vi "Test Queues.vi"() -> ()   [LabVIEW 2019, in "Generator.lvclass"]
uses:
  Generator.lvclass
  typedefs/Waveforms--Cluster.ctl
  <vilib>/measure/NI_MABase.lvlib
panel:
  out "# elements":i32
  out "Waveform Chart":cluster{dbl, dbl}(graph)
  in  "stop":bool
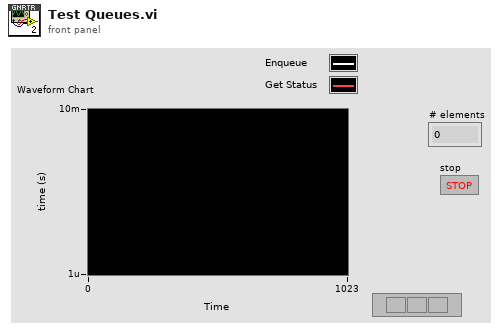
[diagram p1: front panel]
types:
  T1 = typedef "Generator.lvclass/Waveforms--Cluster.ctl" = cluster{"AO":waveform(dbl)[], "REF_X":waveform(dbl)[], "REF_Y":waveform(dbl)[]}
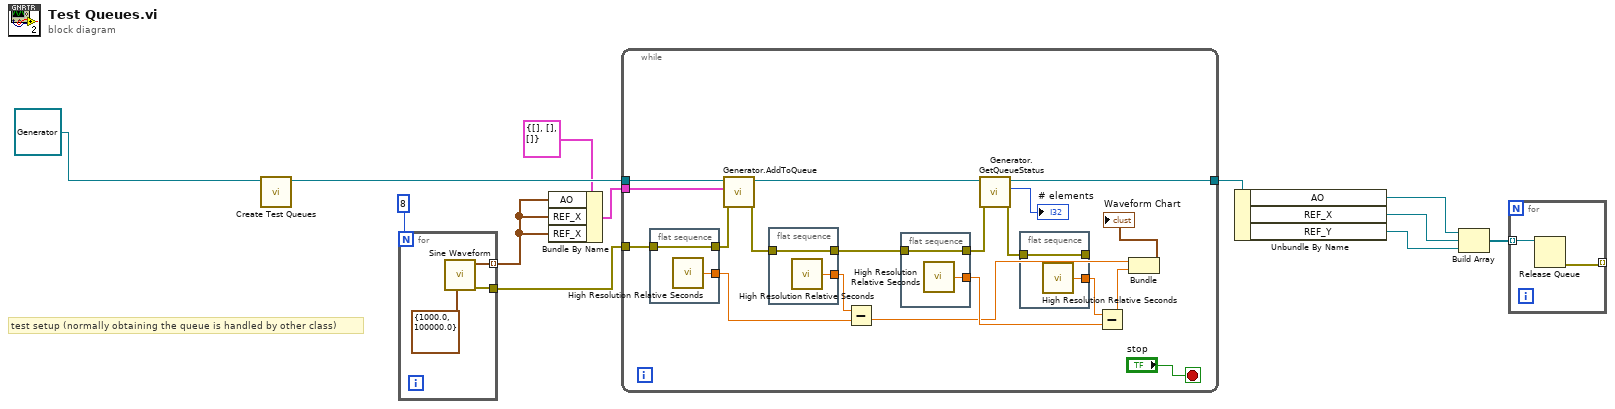
[diagram p0: block diagram]
diagram:
  # "test setup (normally obtaining the queue is handled by other class)"
  n1 = call "Create Test Queues.vi"("Generator in"=refnum<class "Generator.lvclass"> refnum ("Generator.lvclass")) -> ("Generator out"=w12:refnum<class "Generator.lvclass">)  [unwired: 10 in]
  n2 = for {
    N: 8 -> [_]
    tunnel: [w14] -> w7 mode=indexing
    tunnel: [w13] -> w8
    n3 = call <vilib>:"Sine Waveform.vi"("sampling info"=cluster{"Fs":dbl, "#s":dbl} {"Fs"=1000.0, "#s"=100000.0}) -> ("error out"=w13:errorcluster, "signal out"=w14:waveform(dbl))  [unwired: 9 in]
  }
  n4 = Bundle By Name(cluster=T1 {"AO"=[], "REF_X"=[], "REF_Y"=[]} ("Waveforms"), "AO"=w7, "REF_X"=w7, "REF_X"=w7) -> (w10:T1)
  n5 = while {
    tunnel: w12 -> [w34]
    tunnel: w10 -> [w20]
    tunnel: w8 -> [w19]
    tunnel: [w17] -> w6
    stop <- "stop" stop-if-true
    n6 = flat-sequence {
      tunnel: [w42] -> w31
      tunnel: w19 -> [w41]
      tunnel: [w41] -> w29
      frame #0 {
        n7 = call <vilib>:"High Resolution Relative Seconds.vi"() -> ("relative seconds"=w42:dbl)
      }
    }
    n8 = call "Generator.AddToQueue.vi"("error in (no error)"=w29, "Waveforms"=w20, "Generator in"=w34) -> ("error out"=w30:errorcluster, "Generator out"=w33:refnum<class "Generator.lvclass">)  [unwired: 7 in]
    n9 = flat-sequence {
      tunnel: [w40] -> w32
      tunnel: [w39] -> w25
      tunnel: w30 -> [w39]
      frame #0 {
        n10 = call <vilib>:"High Resolution Relative Seconds.vi"() -> ("relative seconds"=w40:dbl)
      }
    }
    n11 = Subtract(x=w32, y=w31) -> (x-y=w21:dbl)
    n12 = flat-sequence {
      tunnel: [w38] -> w27
      tunnel: w25 -> [w37]
      tunnel: [w37] -> w24
      frame #0 {
        n13 = call <vilib>:"High Resolution Relative Seconds.vi"() -> ("relative seconds"=w38:dbl)
      }
    }
    n14 = call "Generator.GetQueueStatus.vi"("error in (no error)"=w24, "Generator in"=w33) -> ("error out"=w23:errorcluster, "# elements"=→"# elements":i32, "Generator out"=w17:refnum<class "Generator.lvclass">)  [unwired: 7 in]
    n15 = flat-sequence {
      tunnel: [w36] -> w26
      tunnel: [w35] -> _
      tunnel: w23 -> [w35]
      frame #0 {
        n16 = call <vilib>:"High Resolution Relative Seconds.vi"() -> ("relative seconds"=w36:dbl)
      }
    }
    n17 = Subtract(x=w26, y=w27) -> (x-y=w22:dbl)
    n18 = Bundle(w21, w22) -> (→"Waveform Chart":cluster{dbl, dbl})  [unwired: 1 in]
  }
  n19 = Unbundle By Name(w6) -> ("AO"=w3:refnum<queue>, "REF_X"=w5:refnum<queue>, "REF_Y"=w4:refnum<queue>)
  n20 = Build Array(w3, w5, w4) -> (w2:refnum<queue>[])
  n21 = for {
    tunnel: w2 -> [w44] mode=indexing
    tunnel: [w43] -> _ mode=indexing
    n22 = Release Queue(queue=w44) -> (error out=w43:errorcluster)  [unwired: 2 in, 2 out]
  }
